vi "Check Status.vi"(8 "error in (no error)":errorcluster, 11 "Synapse CCD in":refnum<class "Synapse CCD.lvclass">) -> (0 "error out":errorcluster, 1 "Status":string, 2 "Ready?":bool, 3 "Synapse CCD out":refnum<class "Synapse CCD.lvclass">)   [LabVIEW 2017, in "Synapse CCD.lvclass"]
doc: "(Dynamic) Check if the instrument is powered on and update its member fields with the instrument's current status. Optionally return a text status message."
uses:
  Synapse CCD.lvclass
  Synapse CCD.lvclass/Synapse CCD.ctl
  Utility Classes/Readable/Readable.lvclass
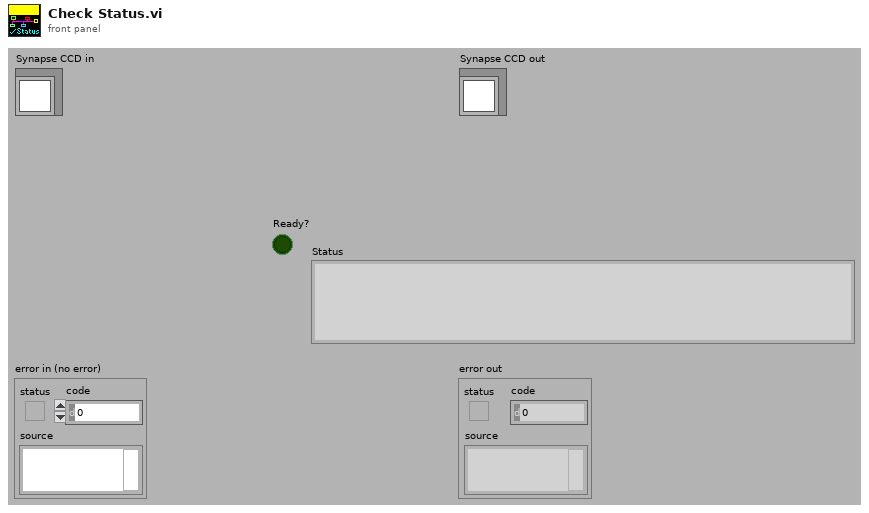
[diagram p1: front panel]
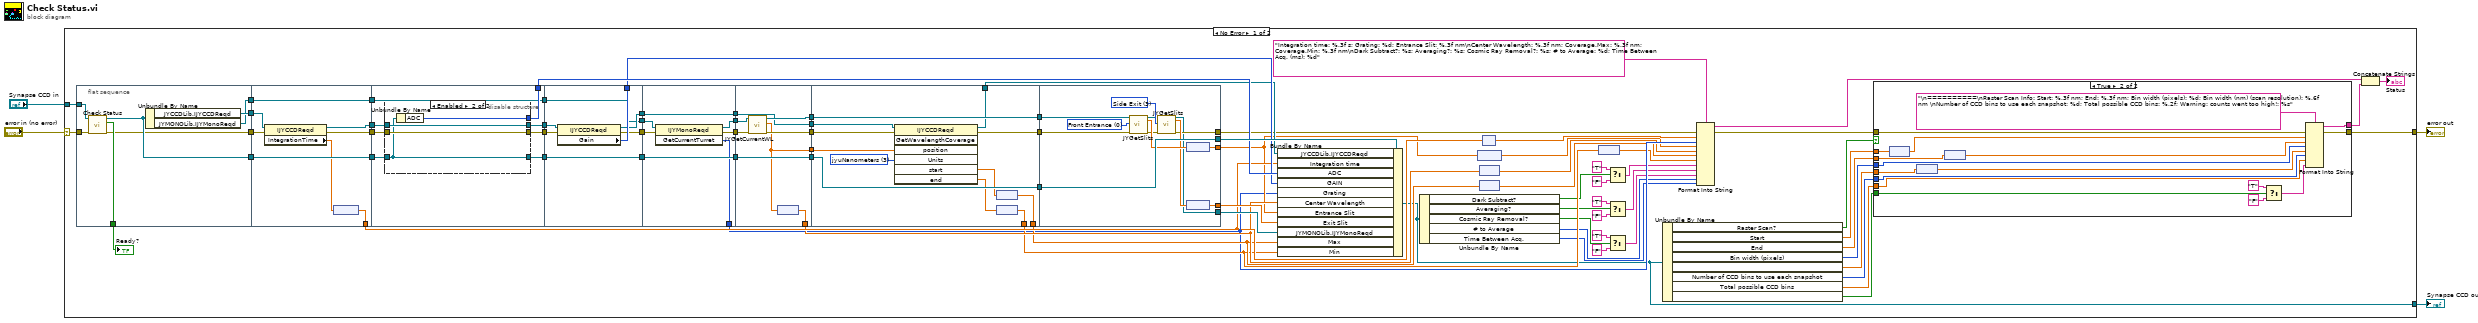
[diagram p0: block diagram]
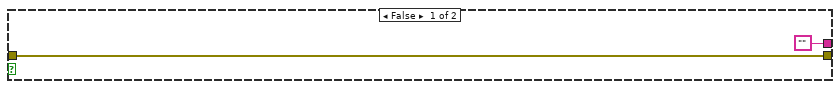
[diagram p2: hidden frame]
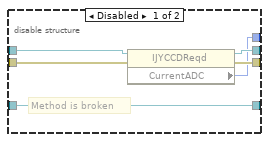
[diagram p3: hidden frame]
diagram:
  n1 = case shown="No Error" "error in (no error)" {
    selector: "error in (no error)" -> [w59 w182]
    tunnel: "Synapse CCD in" -> [w65 w183]
    tunnel: [w18 w183] -> w3
    tunnel: [w8 w182] -> w2
    frame No Error {
      n2 = flat-sequence {
        tunnel: w59 -> [w108]
        tunnel: w65 -> [w107]
        tunnel: [w106] -> w53
        tunnel: [w105] -> w57
        tunnel: [w103] -> w52
        tunnel: [w104] -> w51
        tunnel: [w102] -> w46
        tunnel: [w112] -> w82
        tunnel: w53 -> [w116]
        tunnel: [w116] -> w81
        tunnel: [w113] -> w80
        tunnel: [w114] -> w45
        tunnel: w52 -> [w111]
        tunnel: w51 -> [w110]
        tunnel: [w109] -> w47
        tunnel: w46 -> [w109]
        tunnel: w82 -> [w122]
        tunnel: [w121] -> w79
        tunnel: w81 -> [w119]
        tunnel: [w118] -> w78
        tunnel: w80 -> [w124]
        tunnel: [w123] -> w77
        tunnel: [w120] -> w63
        tunnel: [w117] -> w48
        tunnel: w47 -> [w117]
        tunnel: w79 -> [w139]
        tunnel: w78 -> [w141]
        tunnel: [w141] -> w58
        tunnel: w77 -> [w140]
        tunnel: [w138] -> w62
        tunnel: [w137] -> w56
        tunnel: [w136] -> w55
        tunnel: [w135] -> w49
        tunnel: w48 -> [w135]
        tunnel: w58 -> [w148]
        tunnel: [w146] -> w29
        tunnel: [w148] -> w76
        tunnel: [w147] -> w75
        tunnel: [w145] -> w74
        tunnel: [w143] -> w73
        tunnel: w56 -> [w144]
        tunnel: w55 -> [w143]
        tunnel: w49 -> [w142]
        tunnel: w76 -> [w156]
        tunnel: w75 -> [w155]
        tunnel: w74 -> [w153]
        tunnel: [w150] -> w44
        tunnel: [w156] -> w72
        tunnel: [w154] -> w71
        tunnel: [w152] -> w70
        tunnel: w73 -> [w151]
        tunnel: [w151] -> w69
        tunnel: [w149] -> w54
        tunnel: w72 -> [w168]
        tunnel: [w168] -> w68
        tunnel: w71 -> [w166]
        tunnel: w70 -> [w167]
        tunnel: [w167] -> w67
        tunnel: [w165] -> w66
        tunnel: w69 -> [w164]
        tunnel: [w163] -> w50
        tunnel: [w162] -> w42
        tunnel: [w161] -> w41
        tunnel: w54 -> [w160]
        tunnel: [w181] -> w64
        tunnel: w68 -> [w181]
        tunnel: w67 -> [w178]
        tunnel: [w173] -> w43
        tunnel: [w172] -> w61
        tunnel: [w171] -> w19
        tunnel: [w170] -> w60
        tunnel: w66 -> [w169]
        frame #0 {
          n3 = call-parent "Check Status.vi"("error in (no error)"=w108, "Instrument in"=w107) -> ("error out"=w104:errorcluster, "Ready?"=w105:bool, "Instrument out"=w106:refnum<class "Synapse CCD.lvclass">)  [unwired: 6 in, 1 out]
          n4 = Unbundle By Name(w106) -> ("JYCCDLib.IJYCCDReqd"=w103:refnum<k7>, "JYMONOLib.IJYMonoReqd"=w102:refnum<k7>)
        }
        frame #1 {
          n5 = property class="IJYCCDReqd"(reference=w111, error in=w110) -> (reference out=w113:refnum<k7>, error out=w112:errorcluster, "IntegrationTime"=w115:dbl)
          n6 = node(w115) -> (w114:dbl[unit])
        }
        frame #2 {
          n7 = disable-structure shown="Enabled" {
            disable-tunnel: w124 -> [w130 w134]
            disable-tunnel: [w129 w134] -> w123
            disable-tunnel: w122 -> [w128 w133]
            disable-tunnel: [w127 w133] -> w121
            disable-tunnel: [w126 w131] -> w120
            disable-tunnel: w119 -> [w125 w132]
            disable-tunnel: [w125 w132] -> w118
            frame Disabled {
              # "Method is broken"
              n8 = property class="IJYCCDReqd"(reference=w130, error in=w128) -> (reference out=w129:refnum<k7>, error out=w127:errorcluster, "CurrentADC"=w126:i32)
            }
            frame Enabled {
              n9 = Unbundle By Name(w132) -> ("ADC"=w131:u16)
            }
          }
        }
        frame #3 {
          n10 = property class="IJYCCDReqd"(reference=w140, error in=w139) -> (reference out=w136:refnum<k7>, error out=w137:errorcluster, "Gain"=w138:i32)
        }
        frame #4 {
          n11 = invoke class="IJYMonoReqd" method="GetCurrentTurret"(reference=w142, error in=w144) -> (reference out=w145:refnum<k7>, error out=w147:errorcluster, "GetCurrentTurret"=w146:i32)  [unwired: 1 in]
        }
        frame #5 {
          n12 = call "JYGetCurrentWL.vi"("error in (no error)"=w155, "JYMONOLib.IJYMonoReqd In"=w153) -> ("error out"=w154:errorcluster, "Current WL"=w149:dbl, "JYMONOLib.IJYMonoReqd Out"=w152:refnum<k7>)  [unwired: 6 in, 1 out]
          n13 = node(w149) -> (w150:dbl[unit])
        }
        frame #6 {
          w159 = 3 items=["jyuUndefined", "jyuMillimeters", "jyuMicrons", "jyuNanometers", "jyuAngstroms", "jyuPicometers", "jyuBandpass", "jyuSteps", "jyuWavenumbers", "jyuDeltaWavenumbers", "jyuElectronVolts", "jyuNanoseconds", "jyuMicroseconds", "jyuMilliseconds", "jyuSeconds", "jyuMinutes", "jyuHours", "jyuVolts", "jyuMillivolts", "jyuMicrovolts", "jyuAmperes", "jyuMilliAmps", "jyuMicroAmps", "jyuCounts", "jyuCountsPerSecond", "jyuDegreesCelcius", "jyuDegreesFahrenheit", "jyuDegreesKelvin", "jyuPixels", "jyuTotalUnitsPlusOne"] ("Units")
          n14 = invoke class="IJYCCDReqd" method="GetWavelengthCoverage"(reference=w164, error in=w166, "position"=w160, "Units"=w159) -> (reference out=w163:refnum<k7>, error out=w165:errorcluster, "start"=w158:dbl, "end"=w157:dbl)  [unwired: 3 in, 3 out]
          n15 = node(w158) -> (w162:dbl[unit])
          n16 = node(w157) -> (w161:dbl[unit])
        }
        frame #7 {
          w179 = u16 0 items=["Front Entrance", "Side Entrance", "Front Exit", "Side Exit", "First Intermediate", "Second Intermediate"] ("Slit")
          w180 = u16 3 items=["Front Entrance", "Side Entrance", "Front Exit", "Side Exit", "First Intermediate", "Second Intermediate"] ("Slit")
          n17 = call "JYGetSlits.vi"("MonoRefNum IN"=w178, "Slit"=w179, "error in (no error)"=w169) -> ("MonoRefNum Out"=w175:refnum<k7>, "Slit Width"=w177:dbl, "error out"=w176:errorcluster)  [unwired: 13 in, 1 out]
          n18 = call "JYGetSlits.vi"("MonoRefNum IN"=w175, "Slit"=w180, "error in (no error)"=w176) -> ("MonoRefNum Out"=w170:refnum<k7>, "Slit Width"=w174:dbl, "error out"=w171:errorcluster)  [unwired: 13 in, 1 out]
          n19 = node(w177) -> (w173:dbl[unit])
          n20 = node(w174) -> (w172:dbl[unit])
        }
      }
      n21 = Bundle By Name(cluster=w64, "JYCCDLib.IJYCCDReqd"=w50, "Integration time"=w45, "ADC"=w63, "GAIN"=w62, "Grating"=w29, "Center Wavelength"=w44, "Entrance Slit"=w43, "Exit Slit"=w61, "JYMONOLib.IJYMonoReqd"=w60, "Max"=w42, "Min"=w41) -> (w18:refnum<class "Synapse CCD.lvclass">)
      n22 = Unbundle By Name(w18) -> ("Dark Subtract?"=w40:bool, "Averaging?"=w33:bool, "Cosmic Ray Removal?"=w32:bool, "# to Average"=w21:u32, "Time Between Acq."=w20:u32)
      n23 = node(w43) -> (w28:dbl)
      n24 = node(w44) -> (w27:dbl)
      n25 = node(w42) -> (w26:dbl)
      n26 = node(w45) -> (w30:dbl)
      n27 = node(w41) -> (w25:dbl)
      n28 = Select(t="T", s=w40, f="F") -> (s? t:f=w24:string)
      n29 = Select(t="T", s=w33, f="F") -> (s? t:f=w23:string)
      n30 = Select(t="T", s=w32, f="F") -> (s? t:f=w22:string)
      n31 = Unbundle By Name(w18) -> ("Raster Scan?"=w17:bool, "Start"=w16:dbl[unit], "End"=w15:dbl[unit], "Bin width (pixels)"=w14:i32, "Bin width (nm)\n(scan resolution)"=w13:dbl[unit], "Number of CCD bins to use each snapshot"=w12:i32, "Total possible CCD bins"=w11:dbl, "Warning: counts \nwent too high!"=w10:bool)
      n32 = Format Into String(format string="Integration time: %.3f s; Grating: %d; Entrance Slit: %.3f nm\nCenter Wavelength: %.3f nm; Coverage.Max: %.3f nm; Coverage.Min: %.3f nm\nDark Subtract?: %s; Averaging?: %s; Cosmic Ray Removal?: %s; # to Average: %d; Time Between Acq. (ms): %d", error in=w19, w30, w29, w28, w27, w26, w25, w24, w23, w22, w21, w20) -> (resulting string=w7:string, error out=w9:errorcluster)  [unwired: 1 in]
      n33 = case shown="True" w17 {
        tunnel: w16 -> [_ w98]
        tunnel: w15 -> [_ w97]
        tunnel: w14 -> [_ w89]
        tunnel: w13 -> [_ w96]
        tunnel: w12 -> [_ w87]
        tunnel: w11 -> [_ w86]
        tunnel: w10 -> [_ w95]
        tunnel: w9 -> [w83 w94]
        tunnel: [w83 w93] -> w8
        tunnel: ["" w92] -> w6
        frame False {
        }
        frame True {
          n34 = node(w98) -> (w91:dbl)
          n35 = node(w96) -> (w88:dbl)
          n36 = node(w97) -> (w90:dbl)
          n37 = Select(t="T", s=w95, f="F") -> (s? t:f=w85:string)
          n38 = Format Into String(format string="\n==========\nRaster Scan Info: Start: %.3f nm; End: %.3f nm; Bin width (pixels): %d; Bin width (nm) (scan resolution): %.6f nm \nNumber of CCD bins to use each snapshot: %d; Total possible CCD bins: %.2f; Warning: counts went too high!: %s", error in=w94, w91, w90, w89, w88, w87, w86, w85) -> (resulting string=w92:string, error out=w93:errorcluster)  [unwired: 1 in]
        }
      }
      n39 = Concatenate Strings(w7, w6) -> (→"Status":string)
      "Ready?" <- w57
    }
    frame Error {
    }
  }
  "error out" <- w2
  "Synapse CCD out" <- w3
